vi "1.2.1.5-Gen RW Send Case.vi"(3 "Local Clock: Clk":i8, 4 "Foreign Clock: Clk*":i8, 5 "RS232-1\\Port1 Read Timeout":bool) -> (0 "RS232-1\\Port1 Read":bool, 1 "New Local Clock: Clk":i8, 2 "State":T1(ring))   [LabVIEW 2010]
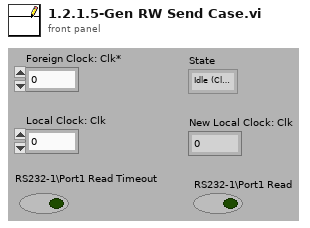
[diagram p1: front panel]
types:
  T1 = enum8{"Idle (Clk=-1)", "Sending(Clk*==Clk+1?Clk=Clk*:;)", "Receiving(Clk*==Clk?Clk++:;)"}
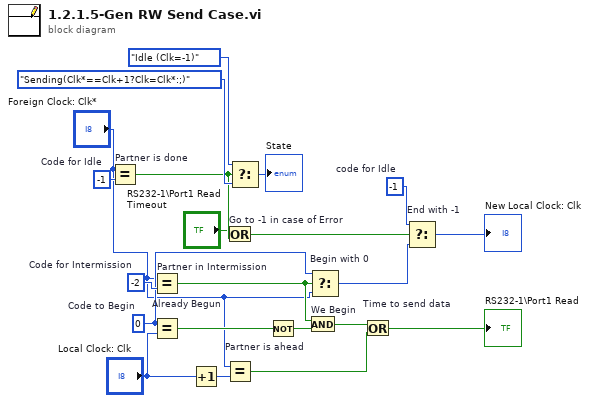
[diagram p0: block diagram]
diagram:
  w14 = i8 -1  # code for Idle
  w16 = i8 -1  # Code for Idle
  w10 = i8 0  # Code to Begin
  w20 = i8 -2  # Code for Intermission
  n1 = Equal? "Partner is done"(x="Foreign Clock: Clk*", y=w16) -> (x = y?=w13:bool)
  n2 = Equal? "Partner in Intermission"(x="Foreign Clock: Clk*", y=w20) -> (x = y?=w7:bool)
  n3 = Equal? "Already Begun"(x=w10, y="Local Clock: Clk") -> (x = y?=w9:bool)
  n4 = Increment(x="Local Clock: Clk") -> (x+1=w5:i8)
  n5 = Or "Go to -1 in case of Error"(x="RS232-1\\Port1 Read Timeout", y=w13) -> (x .or. y?=w12:bool)
  n6 = Equal? "Partner is ahead"(x="Foreign Clock: Clk*", y=w5) -> (x = y?=w2:bool)
  n7 = Select(t=T1."Idle (Clk=-1)", s=w13, f=T1."Sending(Clk*==Clk+1?Clk=Clk*:;)" ("State")) -> (s? t:f=→"State":T1)
  n8 = Not(x=w9) -> (.not. x?=w8:bool)
  n9 = And "We Begin"(x=w7, y=w8) -> (x .and. y?=w3:bool)
  n10 = Select "Begin with 0"(t=w10, s=w7, f="Foreign Clock: Clk*") -> (s? t:f=w19:i8)
  n11 = Or "Time to send data"(x=w3, y=w2) -> (x .or. y?=→"RS232-1\\Port1 Read":bool)
  n12 = Select "End with -1"(t=w14, s=w12, f=w19) -> (s? t:f=→"New Local Clock: Clk":i8)
